vi "Run Tests - When Tests Provided - Returns Test Results For Same Test Cases.vi"(10 "Test Results":refnum<class "Test Result.lvclass">[](array[class]), 11 "Test Cases":refnum<class "Test Case.lvclass">[](array[class])) -> (0 "error out":errorcluster)   [LabVIEW 2017, in "LVUnit Test Executor.Tests.lvlib"]
uses:
  LVUnit Test Executor.Tests.lvlib
  Test Case/Test Case.lvclass
  Test Result/Test Result.lvclass
  LVUnit Test Executor/LVUnit Test Executor.lvclass
  ea609a02-97bf-455b-8325-a132019a9a97.vi
  Constraint/IsEqual/Create.vi
  Constraint/IsEqual/IsEqual.lvclass
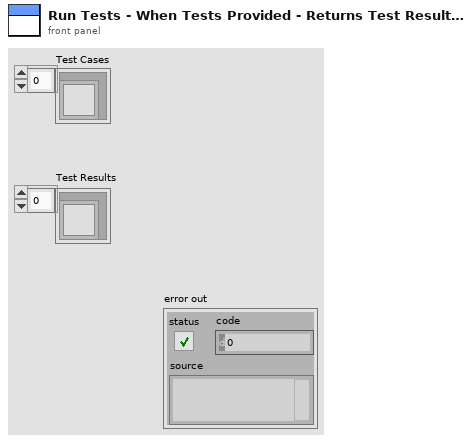
[diagram p1: front panel]
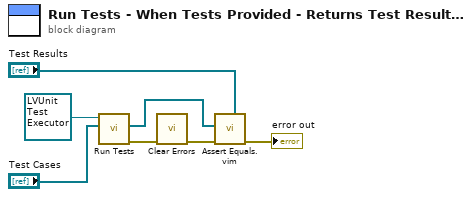
[diagram p0: block diagram]
diagram:
  n1 = call-dynamic "Run Tests.vi"("Test Cases"="Test Cases", "LVUnit Test Executor in"=refnum<class "LVUnit Test Executor.lvclass"> refnum ("LVUnit Test Executor")) -> ("error out"=w5:errorcluster, "Test Results"=w3:refnum<class "Test Result.lvclass">[])  [unwired: 7 in, 1 out]
  n2 = call <vilib>:"Clear Errors.vi"("error in (no error)"=w5) -> ("error out"=w1:errorcluster)  [unwired: 5 in, 1 out]
  n3 = call "Assert Equals.vim"("Expected"="Test Results", "error in (no error)"=w1, "Actual"=w3) -> ("error out"=→"error out":errorcluster)  [unwired: 8 in]
